vi "Ref_Num_Chart_Generation.vi"(0 "error in (no error)":errorcluster, 1 "Type of Chart":u16(ring) items=[" Crude Semi-Log (Short)", "Crude Semi-Log (Long)", "Bi-directional Crude Semi-Log (Short)", "Bi-directional Crude Semi-Log (Long)"], 2 "Polarity for Max Voltage":u16(ring) items=["Positive", "Negative"], 5 "Start":bool, 6 "Max Voltage":dbl, 10 "CGF_Result T.V.":refnum<vi>, 11 "CGF_START":refnum<vi>, 12 "CGF_error in":refnum<vi>, 14 "CGF_error out":refnum<vi>, 15 "CGF_FINISH":refnum<vi>) -> (4 "error out":errorcluster, 7 "~~ FINISH ~~":bool, 9 "Result - Test Voltages Array":dbl[](array[numeric]))   [LabVIEW 2020]
uses:
  Global 1.vi
panel:
  in  "VRmax":dbl
  in  "x":i32
  out "PositiveVoltages[256]":dbl[](array[numeric])
  out "Checking Value of X":i32
  out "UniD : Test Voltages <OUTPUT>":dbl[](array[numeric])
  in  "SUB SCLC":bool
  out "DONE SUB SCLC":bool
  out "UNIDIRECTIONAL - FINISH Formulating Test Voltages":bool
  in  "SUB LCLC":bool
  out "DONE SUB LCLC":bool
  in  "NumberOfVoltages":i32
  out "NegativeVoltages[256]":dbl[](array[numeric])
  out "Negative value":dbl
  out "Crude Semi-Log (Short)":bool
  out "Crude Semi-Log (Long)":bool
  out "Bi-directional Crude Semi-Log (Short)":bool
  out "Bi-directional Crude Semi-Log (Long)":bool
  out "BIDIRECTIONAL = FINISH Formulating Test Voltages":bool
  in  "SUB Bi-SCLC":bool
  in  "SUB Bi-LCLC":bool
  out "DONE SUB Bi-SCLC":bool
  out "DONE SUB Bi-LCLC":bool
  out "Checking NumberOfVoltages":i32
  out "Flag Formula SCLC":bool
  out "Flag Formula LCLC":bool
  out "first subarray : PosTestV":dbl[](array[numeric])
  out "reversed array : NegTestV":dbl[](array[numeric])
  out "BiD : Test Voltages <OUTPUT>":dbl[](array[numeric])
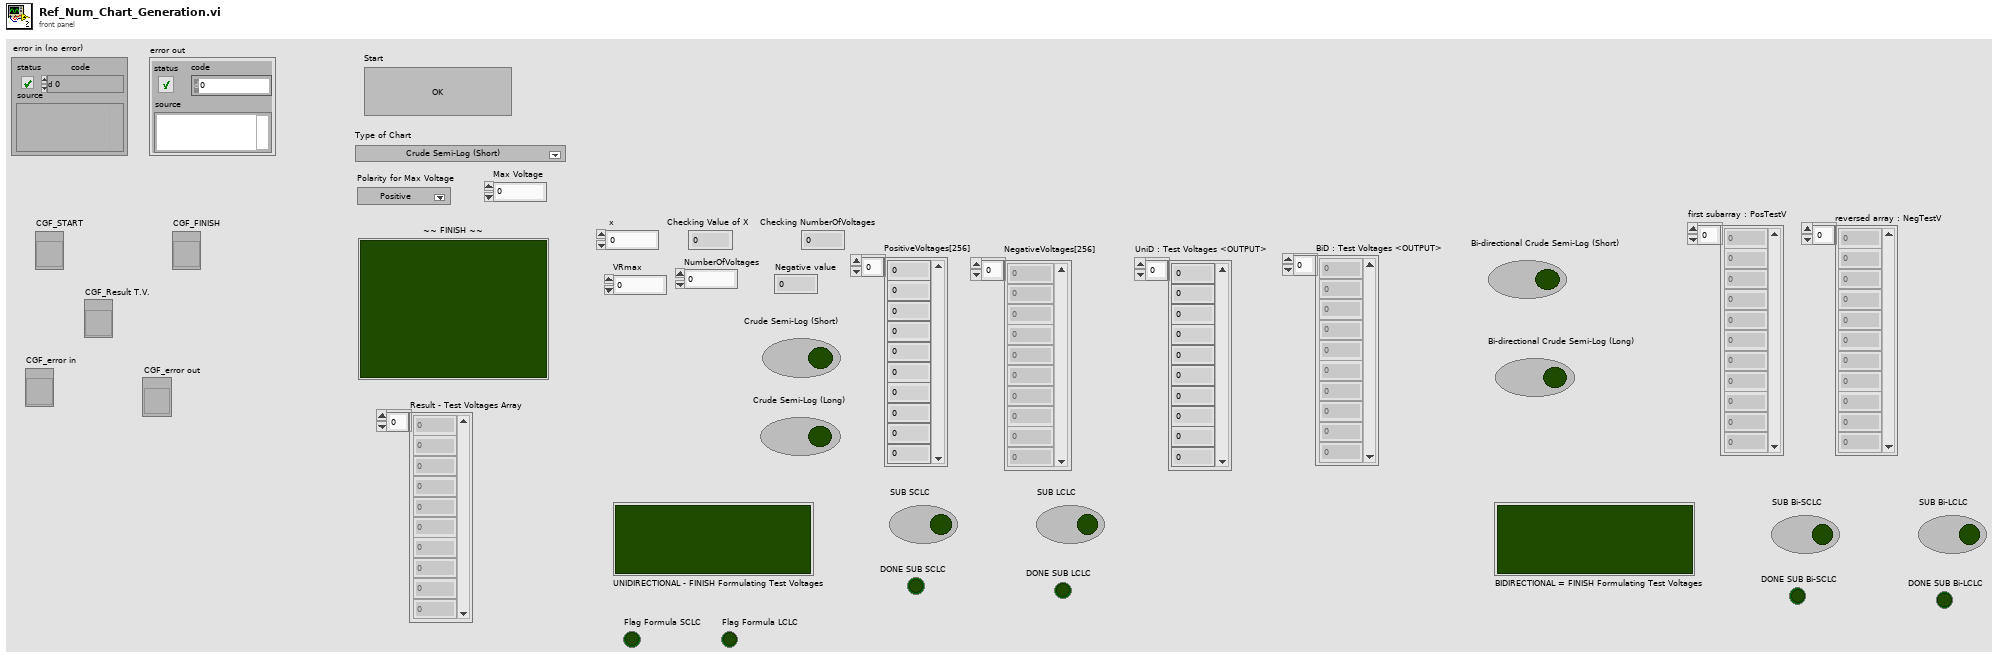
[diagram p1: front panel]
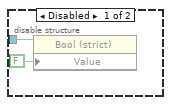
[diagram p2: hidden frame]
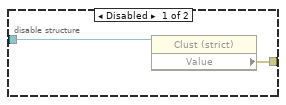
[diagram p3: hidden frame]
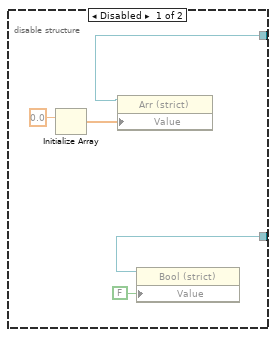
[diagram p4: hidden frame]
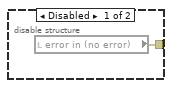
[diagram p5: hidden frame]
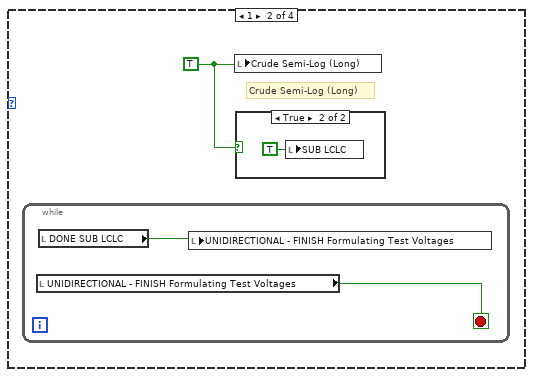
[diagram p7: hidden frame]
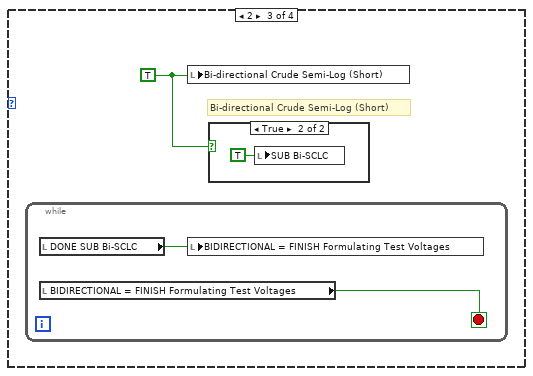
[diagram p9: hidden frame]
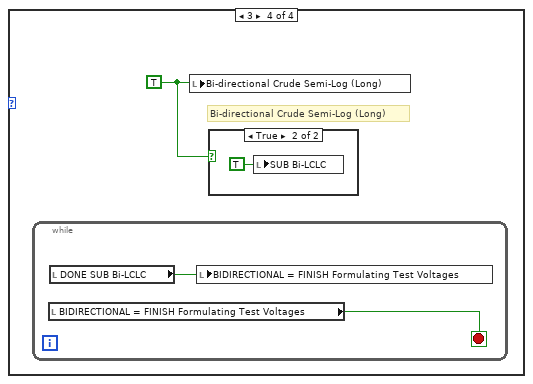
[diagram p11: hidden frame]
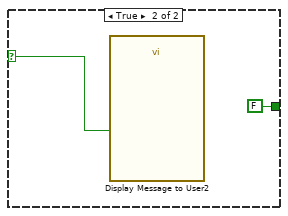
[diagram p16: hidden frame]
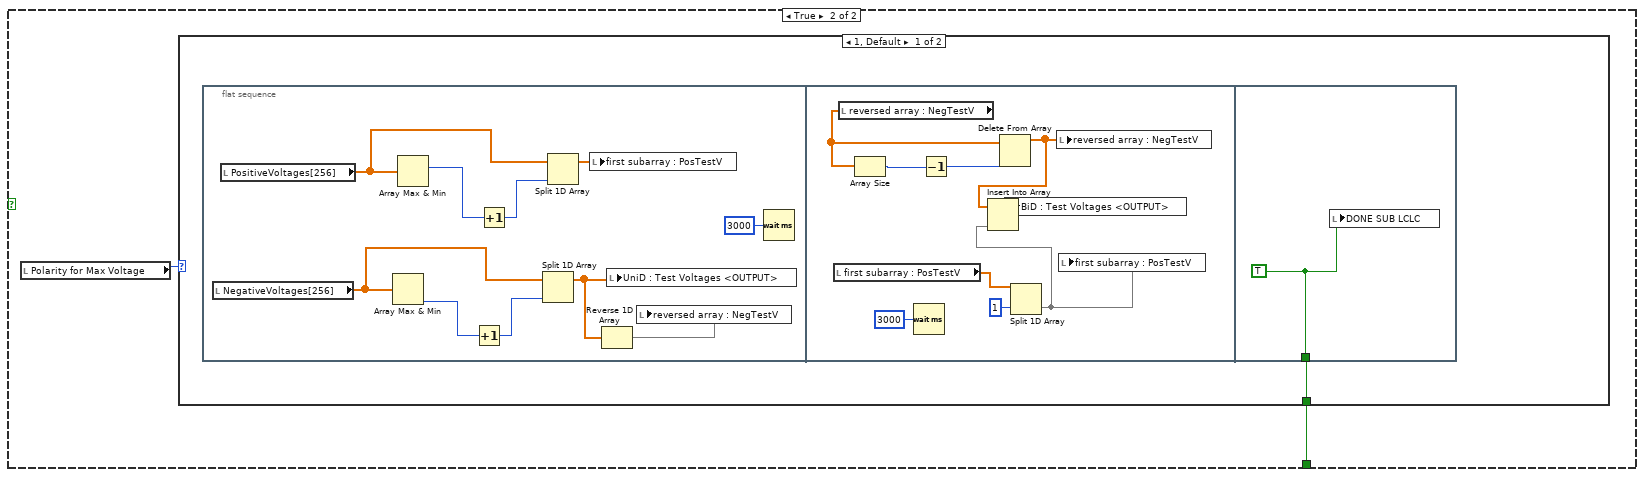
[diagram p17: hidden frame]
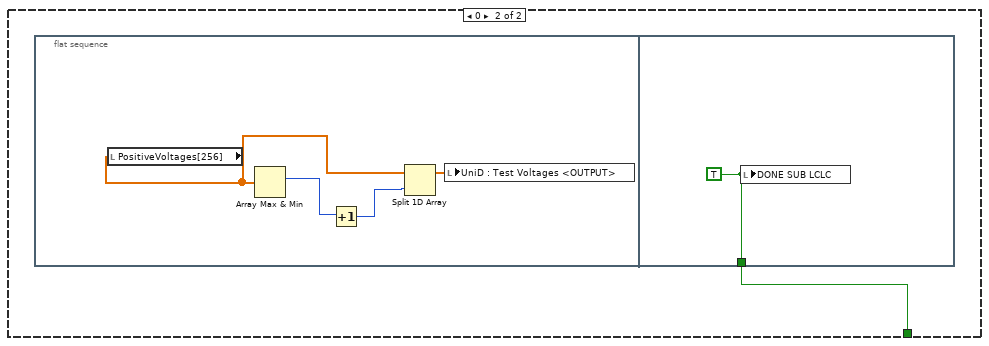
[diagram p18: hidden frame]
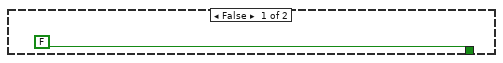
[diagram p19: hidden frame]
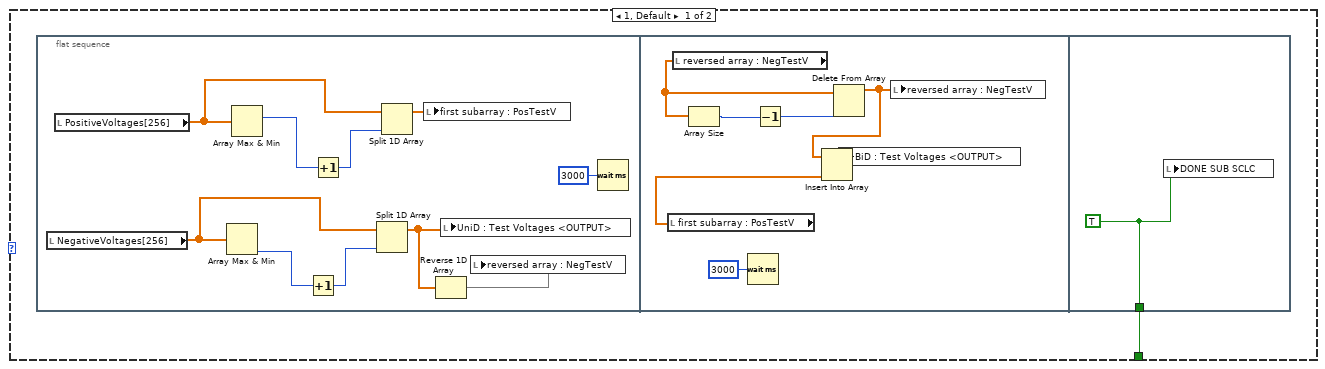
[diagram p20: hidden frame]
diagram:
  n1 = disable-structure shown="Enabled" {
    disable-tunnel: "CGF_error in" -> [w10 _]
    disable-tunnel: "CGF_error out" -> [w9 _]
    disable-tunnel: "CGF_START" -> [w6 _]
    disable-tunnel: "CGF_FINISH" -> [w7 _]
    disable-tunnel: "CGF_Result T.V." -> [w8 _]
    frame Enabled {
      w22 = 0.0
      w11 = FALSE
      # "Bi-directional Crude Semi-Log (Long)"
      # "Bi-directional Crude Semi-Log (Short)"
      # "Initialize"
      # "State Machine of VI"
      # "Error Handler"
      # "Long Sortalog chart bidirectional"
      # "="
      # "Short Sortalog chart bidirectional"
      # "="
      # "="
      # "="
      # "Long Sortalog chart unidirectional"
      # "Short Sortalog chart unidirectional"
      # "Bi-directional Crude Semi-Log (Long)"
      # "Bi-directional Crude Semi-Log (Short)"
      # "Crude Semi-Log (Long)"
      # "Crude Semi-Log (Short)"
      # "DONE :\n\n1) SUB SCLC\n2) SUB SCLC"
      # "ALL VARIABLES"
      # "SUB Function :\nLongCrudeLogChart (VRmax!, Polarity$)"
      # "SUB Function :\n ShortCrudeLogChart (VRmax!, Polarity$)"
      # "Type of Chart :\n\n1) Linear\n2) Crude Semi-Log (Short) \n3) Crude Semi-Log (Long)\n4) Bi-directional Crude Semi-Log (Short)\n5) Bi-directional Crude Semi-Log (Long)"
      # "Linear has been done by Daniel in Generate_Report_NEW\n\nXY Graph : \nArray of X -> Test Voltages\nArray of Y -> Result Arrays"
      n2 = flat-sequence {
        frame #0 {
          n3 = while {
            stop <- w286 stop-if-true
            n4 = local read "SUB SCLC"() -> (w286:bool)
          }
        }
        frame #1 {
          w294 = dbl[] [0.0, 0.1, 0.2, 0.3, 0.4, 0.5, 0.7, 1.0, 2.0, 3.0, 4.0, 5.0, 7.0, 10.0, 20.0, 30.0, 40.0, 50.0, 70.0, 100.0, 200.0]
          # "Bias V"
          n5 = local read "NumberOfVoltages"() -> (w288:i32)
          n6 = Array Max & Min(array=w294) -> (max value=w293:dbl)  [unwired: 3 out]
          n7 = local read "VRmax"() -> (w291:dbl)
          n8 = local read "x"() -> (w292:i32)
          n9 = formula code="// declaration\n\nNumberOfVoltages = 1;\nfloat TestVoltages[256];\n\nx = 1 ;\n//while loop\n\n while   ( VRmax > BiasV[x]  &&  x <= UpBound ) \n {\n\nTestVoltages[x] = BiasV[x];\nx = x + 1;\n}\n//\n\nTestVoltages[x] = VRmax;\nNumberOfVoltages = x;"("x"=w292, "VRmax"=w291, "BiasV"=w294, "NumberOfVoltages"=w288, "UpBound"=w293) -> ("x"=w290:i32, "TestVoltages"=w289:dbl[], "NumberOfVoltages"=w287:i32)
          n10 = local write "PositiveVoltages[256]"(w289) -> ()
          n11 = local write "Checking NumberOfVoltages"(w287) -> ()
          n12 = local write "Checking Value of X"(w290) -> ()
        }
        frame #2 {
          # "If Polarity = 1, then Polarity = Negative"
          # "Create array with negative value for Polarity = Negative"
          n13 = local read "Polarity for Max Voltage"() -> (w295:u16)
          n14 = case shown="0, Default" w295 {
            frame 0, Default {
            }
            frame 1 {
              n15 = local read "PositiveVoltages[256]"() -> (w297:dbl[])
              n16 = Array Size(array=w297) -> (size(s)=w296:i32)
              n17 = for {
                N: w296 -> [_]
                tunnel: w297 -> [w303]
                i -> [w300]
                n18 = Index Array(array=w303, index=w300) -> (element=w304:dbl)
                n19 = Wait (ms)(milliseconds to wait=u32 1000) -> ()  [unwired: 1 out]
                n20 = Negate(x=w304) -> (-x=w301:dbl)
                n21 = local write "Negative value"(w301) -> ()
                n22 = feedback #1() -> (w299:dbl[])  [unwired: 1 in]
                n23 = local write "NegativeVoltages[256]"(w299) -> ()
                n24 = Insert Into Array(array=w299, index=w300, new element=w301) -> (w298:dbl[])
                n25 = feedback-in #1(w298) -> ()
              }
            }
          }
        }
        frame #3 {
          # "Add last element into Negative Array"
          # "If Polarity = 1, then Polarity = Negative"
          n26 = local read "Polarity for Max Voltage"() -> (w305:u16)
          n27 = case shown="0, Default" w305 {
            frame 0, Default {
            }
            frame 1 {
              n28 = local read "NegativeVoltages[256]"() -> (w306:dbl[])
              n29 = Wait (ms)(milliseconds to wait=u32 500) -> ()  [unwired: 1 out]
              n30 = local read "PositiveVoltages[256]"() -> (w309:dbl[])
              n31 = Array Max & Min(array=w309) -> (max index (indices)=w308:i32)  [unwired: 3 out]
              n32 = Index Array(array=w309, index=w308) -> (element=w312:dbl)
              n33 = Negate(x=w312) -> (-x=w310:dbl)
              n34 = local write "Negative value"(w310) -> ()
              n35 = Insert Into Array(array=w306, index=w308, new element=w310) -> (w307:dbl[])
              n36 = local write "NegativeVoltages[256]"(w307) -> ()
            }
          }
        }
        frame #4 {
          # "Replace -0 to 0 in 1st index of array"
          # "If Polarity = 1, then Polarity = Negative"
          n37 = local read "Polarity for Max Voltage"() -> (w313:u16)
          n38 = case shown="0, Default" w313 {
            frame 0, Default {
            }
            frame 1 {
              n39 = local read "NegativeVoltages[256]"() -> (w317:dbl[])
              n40 = Wait (ms)(milliseconds to wait=u32 500) -> ()  [unwired: 1 out]
              n41 = Replace Array Subset(array=w317, new element=0.0 ("new element/subarray"), index=0) -> (w316:dbl[])
              n42 = local write "NegativeVoltages[256]"(w316) -> ()
            }
          }
        }
        frame #5 {
          n43 = local write "Flag Formula SCLC"(TRUE) -> ()
        }
      }
      n44 = while {
        stop <- w162 stop-if-true
        n45 = local read "Flag Formula SCLC"() -> (w163:bool)
        n46 = Wait (ms)(milliseconds to wait=u32 800) -> ()  [unwired: 1 out]
        n47 = case shown="True" w163 {
          tunnel: [FALSE ("FINISH CHART") w166] -> w162
          frame False {
          }
          frame True {
            n48 = local read "Polarity for Max Voltage"() -> (w165:u16)
            n49 = case shown="0" w165 {
              tunnel: [w167 w186] -> w166
              frame 1, Default {
                n50 = flat-sequence {
                  tunnel: [w185] -> w167
                  frame #0 {
                    n51 = local read "NegativeVoltages[256]"() -> (w177:dbl[])
                    n52 = local read "PositiveVoltages[256]"() -> (w171:dbl[])
                    n53 = Array Max & Min(array=w177) -> (min index (indices)=w176:i32)  [unwired: 3 out]
                    n54 = Array Max & Min(array=w171) -> (max index (indices)=w170:i32)  [unwired: 3 out]
                    n55 = Increment(x=w176) -> (x+1=w173:i32)
                    n56 = Increment(x=w170) -> (x+1=w172:i32)
                    n57 = Split 1D Array(array=w177, index=w173) -> (first subarray=w174:dbl[])  [unwired: 1 out]
                    n58 = Split 1D Array(array=w171, index=w172) -> (first subarray=w169:dbl[])  [unwired: 1 out]
                    n59 = local write "first subarray : PosTestV"(w169) -> ()
                    n60 = Reverse 1D Array(array=w174) -> (reversed array=w168:dbl[])
                    n61 = local write "UniD : Test Voltages <OUTPUT>"(w174) -> ()
                    n62 = local write "reversed array : NegTestV"(w168) -> ()
                    n63 = Wait (ms)(milliseconds to wait=u32 3000) -> ()  [unwired: 1 out]
                  }
                  frame #1 {
                    n64 = local read "first subarray : PosTestV"() -> (w184:dbl[])
                    n65 = local read "reversed array : NegTestV"() -> (w182:dbl[])
                    n66 = Array Size(array=w182) -> (size(s)=w181:i32)
                    n67 = Wait (ms)(milliseconds to wait=u32 3000) -> ()  [unwired: 1 out]
                    n68 = Decrement(x=w181) -> (x-1=w180:i32)
                    n69 = Delete From Array(array=w182, index=w180) -> (array with subset deleted=w178:dbl[])  [unwired: 1 in, 1 out]
                    n70 = Insert Into Array(array=w178, new element=w184) -> (w179:dbl[])  [unwired: 1 in]
                    n71 = local write "BiD : Test Voltages <OUTPUT>"(w179) -> ()
                    n72 = local write "reversed array : NegTestV"(w178) -> ()
                  }
                  frame #2 {
                    w185 = TRUE ("FINISH CHART")
                    n73 = local write "DONE SUB SCLC"(w185) -> ()
                  }
                }
              }
              frame 0 {
                n74 = flat-sequence {
                  tunnel: [w191] -> w186
                  frame #0 {
                    n75 = local read "PositiveVoltages[256]"() -> (w188:dbl[])
                    n76 = Array Max & Min(array=w188) -> (max index (indices)=w190:i32)  [unwired: 3 out]
                    n77 = Increment(x=w190) -> (x+1=w189:i32)
                    n78 = Split 1D Array(array=w188, index=w189) -> (first subarray=w187:dbl[])  [unwired: 1 out]
                    n79 = local write "UniD : Test Voltages <OUTPUT>"(w187) -> ()
                  }
                  frame #1 {
                    w191 = TRUE ("FINISH CHART")
                    n80 = local write "DONE SUB SCLC"(w191) -> ()
                  }
                }
              }
            }
          }
        }
      }
      n81 = flat-sequence {
        frame #0 {
          n82 = while {
            stop <- w51 stop-if-true
            n83 = local read "SUB Bi-SCLC"() -> (w51:bool)
          }
        }
        frame #1 {
          w53 = u16 1 items=["Positive", "Negative"] ("Polarity for Max Voltage")
          n84 = local write "Polarity for Max Voltage"(w53) -> ()
          n85 = Wait (ms)(milliseconds to wait=u32 500) -> ()  [unwired: 1 out]
        }
        frame #2 {
          n86 = while {
            stop <- w56 stop-if-true
            n87 = local read "DONE SUB SCLC"() -> (w56:bool)
          }
          n88 = local write "SUB SCLC"(TRUE ("SUB SCLC")) -> ()
          n89 = Wait (ms)(milliseconds to wait=u32 1000) -> ()  [unwired: 1 out]
        }
        frame #3 {
          n90 = local write "DONE SUB Bi-SCLC"(TRUE ("DONE SUB Bi-SCLC")) -> ()
        }
      }
      n91 = while {
        stop <- w118 stop-if-true
        n92 = local read "Max Voltage"() -> (w120:dbl)
        n93 = Equal?(x=w120, y=999.0) -> (x = y?=w123:bool)
        n94 = Equal?(x=w120, y=-999.0) -> (x = y?=w122:bool)
        n95 = Or(x=w123, y=w122) -> (x .or. y?=w119:bool)
        n96 = case shown="False" w119 {
          selector: w119 -> [_ w127]
          tunnel: [TRUE FALSE] -> w118
          frame False {
          }
          frame True {
            n97 = call "Display Message to User2"("Enable"=w127) -> ()  [unwired: 9 in, 2 out]
          }
        }
      }
      n98 = disable-structure shown="Enabled" {
        disable-tunnel: [w43 _] -> _
        frame Disabled {
          n99 = local read "error in (no error)"() -> (w43:errorcluster)
        }
        frame Enabled {
        }
      }
      n100 = disable-structure shown="Enabled" {
        disable-tunnel: w10 -> [w37 _]
        disable-tunnel: [w36 _] -> _
        frame Disabled {
          n101 = property class="Clust (strict)"(reference=w37) -> ("Value"=w36:errorcluster)  [unwired: 1 in, 2 out]
        }
        frame Enabled {
        }
      }
      n102 = flat-sequence {
        tunnel: [w59] -> w33
        tunnel: w6 -> [w58]
        tunnel: [w66] -> w32
        tunnel: w33 -> [w66]
        tunnel: w32 -> [w86]
        tunnel: w9 -> [w91]
        tunnel: w7 -> [w90]
        tunnel: w8 -> [w89]
        frame #0 {
          n103 = while {
            tunnel: [w62] -> w59
            tunnel: w58 -> [w61]
            stop <- w64 stop-if-true
            n104 = local read "error in (no error)"() -> (w60:errorcluster)
            n105 = property class="Bool (strict)"(reference=w61, error in=w60) -> (error out=w62:errorcluster, "Value"=w63:bool)  [unwired: 1 out]
            n106 = local read "Start"() -> (w65:bool)
            n107 = Or(x=w65, y=w63) -> (x .or. y?=w64:bool)
          }
        }
        frame #1 {
          n108 = local read "Type of Chart"() -> (w69:u16)
          n109 = case shown="0, Default" w69 {
            frame 0, Default {
              w70 = TRUE ("Crude Semi-Log (Short)")
              # "Crude Semi-Log (Short)"
              n110 = while {
                stop <- w71 stop-if-true
                n111 = local read "DONE SUB SCLC"() -> (w72:bool)
                n112 = local read "UNIDIRECTIONAL - FINISH Formulating Test Voltages"() -> (w71:bool)
                n113 = local write "UNIDIRECTIONAL - FINISH Formulating Test Voltages"(w72) -> ()
              }
              n114 = local write "Crude Semi-Log (Short)"(w70) -> ()
              n115 = case shown="True" w70 {
                frame False {
                }
                frame True {
                  n116 = local write "SUB SCLC"(TRUE ("SUB SCLC")) -> ()
                }
              }
            }
            frame 1 {
              w74 = TRUE ("Crude Semi-Log (Long)")
              # "Crude Semi-Log (Long)"
              n117 = while {
                stop <- w75 stop-if-true
                n118 = local read "UNIDIRECTIONAL - FINISH Formulating Test Voltages"() -> (w75:bool)
                n119 = local read "DONE SUB LCLC"() -> (w76:bool)
                n120 = local write "UNIDIRECTIONAL - FINISH Formulating Test Voltages"(w76) -> ()
              }
              n121 = local write "Crude Semi-Log (Long)"(w74) -> ()
              n122 = case shown="True" w74 {
                frame False {
                }
                frame True {
                  n123 = local write "SUB LCLC"(TRUE ("SUB SCLC")) -> ()
                }
              }
            }
            frame 2 {
              w78 = TRUE ("Bi-directional Crude Semi-Log (Short)")
              # "Bi-directional Crude Semi-Log (Short)"
              n124 = while {
                stop <- w79 stop-if-true
                n125 = local read "DONE SUB Bi-SCLC"() -> (w80:bool)
                n126 = local read "BIDIRECTIONAL = FINISH Formulating Test Voltages"() -> (w79:bool)
                n127 = local write "BIDIRECTIONAL = FINISH Formulating Test Voltages"(w80) -> ()
              }
              n128 = local write "Bi-directional Crude Semi-Log (Short)"(w78) -> ()
              n129 = case shown="True" w78 {
                frame False {
                }
                frame True {
                  n130 = local write "SUB Bi-SCLC"(TRUE ("SUB Bi-SCLC")) -> ()
                }
              }
            }
            frame 3 {
              w82 = TRUE ("Bi-directional Crude Semi-Log (Long)")
              # "Bi-directional Crude Semi-Log (Long)"
              n131 = while {
                stop <- w83 stop-if-true
                n132 = local read "BIDIRECTIONAL = FINISH Formulating Test Voltages"() -> (w83:bool)
                n133 = local read "DONE SUB Bi-LCLC"() -> (w84:bool)
                n134 = local write "BIDIRECTIONAL = FINISH Formulating Test Voltages"(w84) -> ()
              }
              n135 = local write "Bi-directional Crude Semi-Log (Long)"(w82) -> ()
              n136 = case shown="True" w82 {
                frame False {
                }
                frame True {
                  n137 = local write "SUB Bi-LCLC"(TRUE ("SUB Bi-LCLC")) -> ()
                }
              }
            }
          }
          n138 = call "Display Message to User3"("Message"="<<  START   >>\nInserting Test Voltages") -> ()  [unwired: 9 in, 2 out]
          n139 = Wait (ms)(milliseconds to wait=u32 1000) -> ()  [unwired: 1 out]
        }
        frame #2 {
          n140 = Wait (ms)(milliseconds to wait=u32 800) -> ()  [unwired: 1 out]
          n141 = while {
            tunnel: [w109] -> w93
            tunnel: w89 -> [w106]
            tunnel: [w103] -> w88
            tunnel: w86 -> [w102]
            tunnel: w86 -> [w101]
            stop <- w109 stop-if-true
            n142 = local read "BIDIRECTIONAL = FINISH Formulating Test Voltages"() -> (w107:bool)
            n143 = local read "UNIDIRECTIONAL - FINISH Formulating Test Voltages"() -> (w108:bool)
            n144 = case shown="True" w108 {
              tunnel: w106 -> [_ w117]
              tunnel: [_ w116] -> w105
              tunnel: w102 -> [_ w115]
              frame False {
              }
              frame True {
                n145 = local read "UniD : Test Voltages <OUTPUT>"() -> (w114:dbl[])
                n146 = global write "Global 1.vi" "Result - Test Voltages Array"(w114) -> ()
                n147 = local write "Result - Test Voltages Array"(w114) -> ()
                n148 = property class="Arr (strict)"(reference=w117, error in=w115, "Value"=w114) -> (error out=w116:errorcluster)  [unwired: 1 out]
              }
            }
            n149 = case shown="True" w107 {
              tunnel: w106 -> [_ w113]
              tunnel: [_ w112] -> w104
              tunnel: w101 -> [_ w111]
              frame False {
              }
              frame True {
                n150 = local read "BiD : Test Voltages <OUTPUT>"() -> (w110:dbl[])
                n151 = local write "Result - Test Voltages Array"(w110) -> ()
                n152 = global write "Global 1.vi" "Result - Test Voltages Array"(w110) -> ()
                n153 = property class="Arr (strict)"(reference=w113, error in=w111, "Value"=w110) -> (error out=w112:errorcluster)  [unwired: 1 out]
              }
            }
            n154 = Or(x=w108, y=w107) -> (x .or. y?=w109:bool)
            n155 = Merge Errors(w105, w104) -> (w103:errorcluster)
          }
          n156 = Merge Errors(w88, w86) -> (w87:errorcluster)
          n157 = case shown="True" w93 {
            selector: w93 -> [_ w98]
            tunnel: w87 -> [_ w97]
            tunnel: w91 -> [_ w99]
            tunnel: w90 -> [_ w96]
            frame False {
            }
            frame True {
              n158 = property class="Bool (strict)"(reference=w96, error in=w97, "Value"=w98) -> (error out=w95:errorcluster)  [unwired: 1 out]
              n159 = property class="Clust (strict)"(reference=w99, error in=w95, "Value"=w95) -> (error out=w94:errorcluster)  [unwired: 1 out]
              n160 = local write "~~ FINISH ~~"(w98) -> ()
              n161 = local write "error out"(w94) -> ()
              n162 = call "Display Message to User4"("Enable"=w98, "Message"="<<  DONE  >> \nInserting Test Voltages") -> ()  [unwired: 8 in, 2 out]
            }
          }
        }
      }
      n163 = disable-structure shown="Enabled" {
        disable-tunnel: w6 -> [w35 _]
        frame Disabled {
          n164 = property class="Bool (strict)"(reference=w35, "Value"=FALSE) -> ()  [unwired: 1 in, 2 out]
        }
        frame Enabled {
        }
      }
      n165 = flat-sequence {
        frame #0 {
          n166 = while {
            stop <- w192 stop-if-true
            n167 = local read "SUB LCLC"() -> (w192:bool)
          }
        }
        frame #1 {
          n168 = local read "VRmax"() -> (w194:dbl)
          n169 = Less Or Equal?(x=w194, y=200.0) -> (x <= y?=w195:bool)
          n170 = case shown="True" w195 {
            frame False {
              n171 = Initialize Array(0.0 ("element")) -> (w197:dbl[])  [unwired: 1 in]
              n172 = local write "PositiveVoltages[256]"(w197) -> ()
              n173 = local write "NumberOfVoltages"(1 ("NumberOfVoltages")) -> ()
            }
            frame True {
              n174 = local read "NumberOfVoltages"() -> (w201:i32)
              n175 = local read "VRmax"() -> (w204:dbl)
              n176 = local read "x"() -> (w202:i32)
              n177 = Multiply(x=w204, y=10.0) -> (x*y=w206:dbl)
              n178 = case shown="0..31" w206 {
                tunnel: w204 -> [w213 w217 w225 w232 w239 w246 w253 _]
                tunnel: [w212 w219 w224 w231 w238 w245 w252 _] -> w203
                tunnel: w202 -> [w211 w218 w226 w233 w240 w247 w254 _]
                tunnel: w201 -> [w210 w220 w227 w234 w241 w248 w255 _]
                tunnel: [w208 w215 w222 w229 w236 w243 w250 _] -> w200
                tunnel: [w207 w214 w221 w228 w235 w242 w249 _] -> w199
                frame 0..31 {
                  n179 = formula code="// declaration\n//' Set bias 0 to VRmax! at 0.1V increments (32 voltages)\nNumberOfVoltages = 1;\nfloat TestVoltages[256];\n\nfor (    (x = 0); (x <= VRmax*10); x++   ){\nTestVoltages[x+1] = x / 10;\nNumberOfVoltages = x + 1;\n}"("VRmax"=w213, "x"=w211, "NumberOfVoltages"=w210) -> ("TestVoltages"=w212:dbl[], "x"=w208:i32, "NumberOfVoltages"=w207:i32)
                  n180 = Wait (ms)(milliseconds to wait=u32 500) -> ()  [unwired: 1 out]
                }
                frame 32..100 {
                  n181 = formula code="// declaration\n//'  Set bias 0,.1,.2,.3,.4,.5,.6,.7,.8,.9,1,1.1,1.2,1.5,2,2.5,...s)\nNumberOfVoltages = 1;\nfloat TestVoltages[256];\n//---------------------------------------------\n//---------------------------------------------\nfor (    (x = 0); (x <=11); x++   ){\nTestVoltages[x+1] = x / 10;\n}\n//---------------------------------------------\nTestVoltages[13] = 1.3;\nTestVoltages[14] = 1.5;\n//---------------------------------------------\nfor (    (x = 4); (x <= VRmax*2); x++   ){\nTestVoltages[11+x] = x / 2;\nNumberOfVoltages =11+x;\n}\n//---------------------------------------------\nTestVoltages[NumberOfVoltages] = abs(VRmax);"("VRmax"=w217, "x"=w218, "NumberOfVoltages"=w220) -> ("TestVoltages"=w219:dbl[], "x"=w215:i32, "NumberOfVoltages"=w214:i32)
                  n182 = Wait (ms)(milliseconds to wait=u32 500) -> ()  [unwired: 1 out]
                }
                frame 101..199 {
                  n183 = formula code="// declaration\n//'  Set bias 0,.1,.2,.3,.4,.5,.6,.7,.8,.9,1,1.1,1.3,1.5,2,3,...\nNumberOfVoltages = 1;\nfloat TestVoltages[256];\n//---------------------------------------------\n//---------------------------------------------\nfor (    (x = 0); (x <=11); x++   ){\nTestVoltages[x+1] = x / 10;\n}\n//---------------------------------------------\nTestVoltages[13] = 1.3;\nTestVoltages[14] = 1.5;\n//---------------------------------------------\nfor (    (x = 2); (x <= int(VRmax)); x++   ){\nTestVoltages[13+x] = x;\nNumberOfVoltages =13+x;\n}\n//---------------------------------------------\nTestVoltages[NumberOfVoltages] = abs(VRmax);"("VRmax"=w225, "x"=w226, "NumberOfVoltages"=w227) -> ("TestVoltages"=w224:dbl[], "x"=w222:i32, "NumberOfVoltages"=w221:i32)
                  n184 = Wait (ms)(milliseconds to wait=u32 500) -> ()  [unwired: 1 out]
                }
                frame 200..300 {
                  n185 = formula code="// declaration\n//'  Set bias 0,.1,.2,.3,.4,.5,.6,.7,.8,.9,1,1.1,1.3,1.5,2,3,...\nNumberOfVoltages = 1;\nfloat TestVoltages[256];\n//---------------------------------------------\n//---------------------------------------------\nfor (    (x = 0); (x<=11); x++   ){\nTestVoltages[x+1] = x / 10;\n}\n//---------------------------------------------\nTestVoltages[13] = 1.3;\nTestVoltages[14] = 1.5;\n//---------------------------------------------\nfor (    (x = 2); (x <= int(VRmax)); x=x+2   ){\nTestVoltages[14+ x/2] = x;\nNumberOfVoltages =14+ x/2;\n}\n//---------------------------------------------\nTestVoltages[NumberOfVoltages] = abs(VRmax);"("VRmax"=w232, "x"=w233, "NumberOfVoltages"=w234) -> ("TestVoltages"=w231:dbl[], "x"=w229:i32, "NumberOfVoltages"=w228:i32)
                  n186 = Wait (ms)(milliseconds to wait=u32 500) -> ()  [unwired: 1 out]
                }
                frame 301..350 {
                  n187 = formula code="// declaration\n//'  Set bias 0,.1,.2,.3,.4,.5,.6,.7,.8,.9,1,1.1,1.3,1.5,2,5,10,...\nNumberOfVoltages = 1;\nfloat TestVoltages[256];\n//---------------------------------------------\n//---------------------------------------------\nfor (    (x = 0); (x <=11); x++   ){\nTestVoltages[x+1] = x / 10;\n}\n//---------------------------------------------\nTestVoltages[13] = 1.3;\nTestVoltages[14] = 1.5;\nTestVoltages[15] = 2;\n//---------------------------------------------\nfor (    (x =5); (x <= int(VRmax)); x=x+5   ){\nTestVoltages[15+ x/5] = x;\nNumberOfVoltages =15+ x/5;\n}\n//---------------------------------------------\nTestVoltages[NumberOfVoltages] = abs(VRmax);"("VRmax"=w239, "x"=w240, "NumberOfVoltages"=w241) -> ("TestVoltages"=w238:dbl[], "x"=w236:i32, "NumberOfVoltages"=w235:i32)
                  n188 = Wait (ms)(milliseconds to wait=u32 500) -> ()  [unwired: 1 out]
                }
                frame 351..1000 {
                  n189 = Wait (ms)(milliseconds to wait=u32 500) -> ()  [unwired: 1 out]
                  n190 = formula code="// declaration\n//'  Set bias 0,.1,.2,.3,.4,.5,.6,.7,.8,.9,1,1.1,1.3,1.5,2,5,10,...\nNumberOfVoltages = 1;\nfloat TestVoltages[256];\n//---------------------------------------------\n//---------------------------------------------\nfor (    (x = 0); (x <=11); x++   ){\nTestVoltages[x+1] = x / 10;\n}\n//---------------------------------------------\nTestVoltages[13] = 1.3;\nTestVoltages[14] = 1.5;\nTestVoltages[15] = 2;\nTestVoltages[16] = 5;\nTestVoltages[17] = 10;\n//---------------------------------------------\nfor (    (x =20); (x <= int(VRmax)); x=x+10  ){\nTestVoltages[16+ x/10] = x;\nNumberOfVoltages =16+ x/10;\n}\n//---------------------------------------------\nTestVoltages[NumberOfVoltages] = abs(VRmax);"("VRmax"=w246, "x"=w247, "NumberOfVoltages"=w248) -> ("TestVoltages"=w245:dbl[], "x"=w243:i32, "NumberOfVoltages"=w242:i32)
                }
                frame 1001..2000 {
                  n191 = Wait (ms)(milliseconds to wait=u32 500) -> ()  [unwired: 1 out]
                  n192 = formula code="// declaration\n//'  Set bias 0,.1,.2,.3,.4,.5,.6,.7,.8,.9,1,1.1,1.3,1.5,2,5,10,...\nNumberOfVoltages = 1;\nfloat TestVoltages[256];\n//---------------------------------------------\n//---------------------------------------------\nfor (    (x = 0); (x <=11); x++   ){\nTestVoltages[x+1] = x / 10;\n}\n//---------------------------------------------\nTestVoltages[13] = 1.3;\nTestVoltages[14] = 1.5;\nTestVoltages[15] = 2;\nTestVoltages[16] = 5;\nTestVoltages[17] = 10;\nTestVoltages[18] = 20;\n//---------------------------------------------\nfor (    (x =20); (x <= int(VRmax)); x=x+20  ){\nTestVoltages[17+ x/20] = x;\nNumberOfVoltages =17+ x/20;\n}\n//---------------------------------------------\nTestVoltages[NumberOfVoltages] = abs(VRmax);"("VRmax"=w253, "x"=w254, "NumberOfVoltages"=w255) -> ("TestVoltages"=w252:dbl[], "x"=w250:i32, "NumberOfVoltages"=w249:i32)
                }
                frame 2001.., Default {
                  n193 = call "Display Message to User"() -> ()  [unwired: 10 in, 2 out]
                }
              }
              n194 = local write "PositiveVoltages[256]"(w203) -> ()
              n195 = local write "Checking NumberOfVoltages"(w199) -> ()
              n196 = local write "Checking Value of X"(w200) -> ()
            }
          }
        }
        frame #2 {
          # "If Polarity = 1, then Polarity = Negative"
          # "Create array with negative value for Polarity = Negative"
          n197 = local read "Polarity for Max Voltage"() -> (w256:u16)
          n198 = case shown="1" w256 {
            frame 0, Default {
            }
            frame 1 {
              n199 = local read "PositiveVoltages[256]"() -> (w258:dbl[])
              n200 = Array Size(array=w258) -> (size(s)=w257:i32)
              n201 = for {
                N: w257 -> [_]
                tunnel: w258 -> [w264]
                i -> [w262]
                n202 = Index Array(array=w264, index=w262) -> (element=w265:dbl)
                n203 = Wait (ms)(milliseconds to wait=u32 1000) -> ()  [unwired: 1 out]
                n204 = Negate(x=w265) -> (-x=w259:dbl)
                n205 = local write "Negative value"(w259) -> ()
                n206 = feedback #2() -> (w260:dbl[])  [unwired: 1 in]
                n207 = local write "NegativeVoltages[256]"(w260) -> ()
                n208 = Insert Into Array(array=w260, index=w262, new element=w259) -> (w261:dbl[])
                n209 = feedback-in #2(w261) -> ()
              }
            }
          }
        }
        frame #3 {
          # "Add last element into Negative Array"
          # "If Polarity = 1, then Polarity = Negative"
          n210 = local read "Polarity for Max Voltage"() -> (w266:u16)
          n211 = case shown="1" w266 {
            frame 0, Default {
            }
            frame 1 {
              n212 = local read "NegativeVoltages[256]"() -> (w267:dbl[])
              n213 = Wait (ms)(milliseconds to wait=u32 500) -> ()  [unwired: 1 out]
              n214 = local read "PositiveVoltages[256]"() -> (w270:dbl[])
              n215 = Array Max & Min(array=w270) -> (max index (indices)=w269:i32)  [unwired: 3 out]
              n216 = Index Array(array=w270, index=w269) -> (element=w273:dbl)
              n217 = Negate(x=w273) -> (-x=w271:dbl)
              n218 = local write "Negative value"(w271) -> ()
              n219 = Insert Into Array(array=w267, index=w269, new element=w271) -> (w268:dbl[])
              n220 = local write "NegativeVoltages[256]"(w268) -> ()
            }
          }
        }
        frame #4 {
          # "Delete first Zero in Both of the Array"
          # "If Polarity = 1, then Polarity = Negative"
          n221 = local read "Polarity for Max Voltage"() -> (w274:u16)
          n222 = case shown="1" w274 {
            frame 0, Default {
            }
            frame 1 {
              n223 = local read "NegativeVoltages[256]"() -> (w277:dbl[])
              n224 = Wait (ms)(milliseconds to wait=u32 500) -> ()  [unwired: 1 out]
              n225 = Delete From Array(array=w277, index=0) -> (array with subset deleted=w276:dbl[])  [unwired: 1 in, 1 out]
              n226 = local write "NegativeVoltages[256]"(w276) -> ()
            }
          }
        }
        frame #5 {
          # "Replace -0 to 0 in 1st index of array"
          # "If Polarity = 1, then Polarity = Negative"
          n227 = local read "Polarity for Max Voltage"() -> (w279:u16)
          n228 = case shown="1" w279 {
            frame 0, Default {
            }
            frame 1 {
              n229 = local read "NegativeVoltages[256]"() -> (w283:dbl[])
              n230 = Wait (ms)(milliseconds to wait=u32 500) -> ()  [unwired: 1 out]
              n231 = Replace Array Subset(array=w283, new element=0.0 ("new element/subarray"), index=0) -> (w282:dbl[])
              n232 = local write "NegativeVoltages[256]"(w282) -> ()
            }
          }
        }
        frame #6 {
          n233 = local write "Flag Formula LCLC"(TRUE ("DONE SUB LCLC")) -> ()
        }
      }
      n234 = while {
        stop <- w129 stop-if-true
        n235 = local read "Flag Formula LCLC"() -> (w130:bool)
        n236 = Wait (ms)(milliseconds to wait=u32 800) -> ()  [unwired: 1 out]
        n237 = case shown="False" w130 {
          tunnel: [FALSE ("FINISH CHART") w133] -> w129
          frame False {
          }
          frame True {
            n238 = local read "Polarity for Max Voltage"() -> (w132:u16)
            n239 = case shown="1, Default" w132 {
              tunnel: [w134 w155] -> w133
              frame 1, Default {
                n240 = flat-sequence {
                  tunnel: [w154] -> w134
                  frame #0 {
                    n241 = local read "NegativeVoltages[256]"() -> (w144:dbl[])
                    n242 = local read "PositiveVoltages[256]"() -> (w138:dbl[])
                    n243 = Array Max & Min(array=w144) -> (min index (indices)=w143:i32)  [unwired: 3 out]
                    n244 = Array Max & Min(array=w138) -> (max index (indices)=w137:i32)  [unwired: 3 out]
                    n245 = Increment(x=w143) -> (x+1=w140:i32)
                    n246 = Increment(x=w137) -> (x+1=w139:i32)
                    n247 = Split 1D Array(array=w144, index=w140) -> (first subarray=w141:dbl[])  [unwired: 1 out]
                    n248 = Split 1D Array(array=w138, index=w139) -> (first subarray=w136:dbl[])  [unwired: 1 out]
                    n249 = local write "first subarray : PosTestV"(w136) -> ()
                    n250 = Reverse 1D Array(array=w141) -> (reversed array=w135:dbl[])
                    n251 = local write "UniD : Test Voltages <OUTPUT>"(w141) -> ()
                    n252 = local write "reversed array : NegTestV"(w135) -> ()
                    n253 = Wait (ms)(milliseconds to wait=u32 3000) -> ()  [unwired: 1 out]
                  }
                  frame #1 {
                    n254 = local read "first subarray : PosTestV"() -> (w147:dbl[])
                    n255 = local read "reversed array : NegTestV"() -> (w152:dbl[])
                    n256 = Array Size(array=w152) -> (size(s)=w151:i32)
                    n257 = Wait (ms)(milliseconds to wait=u32 3000) -> ()  [unwired: 1 out]
                    n258 = Decrement(x=w151) -> (x-1=w150:i32)
                    n259 = Delete From Array(array=w152, index=w150) -> (array with subset deleted=w148:dbl[])  [unwired: 1 in, 1 out]
                    n260 = Split 1D Array(array=w147, index=1) -> (second subarray=w145:dbl[])  [unwired: 1 out]
                    n261 = Insert Into Array(array=w148, new element=w145) -> (w149:dbl[])  [unwired: 1 in]
                    n262 = local write "BiD : Test Voltages <OUTPUT>"(w149) -> ()
                    n263 = local write "reversed array : NegTestV"(w148) -> ()
                    n264 = local write "first subarray : PosTestV"(w145) -> ()
                  }
                  frame #2 {
                    w154 = TRUE ("FINISH CHART")
                    n265 = local write "DONE SUB LCLC"(w154) -> ()
                  }
                }
              }
              frame 0 {
                n266 = flat-sequence {
                  tunnel: [w160] -> w155
                  frame #0 {
                    n267 = local read "PositiveVoltages[256]"() -> (w157:dbl[])
                    n268 = Array Max & Min(array=w157) -> (max index (indices)=w159:i32)  [unwired: 3 out]
                    n269 = Increment(x=w159) -> (x+1=w158:i32)
                    n270 = Split 1D Array(array=w157, index=w158) -> (first subarray=w156:dbl[])  [unwired: 1 out]
                    n271 = local write "UniD : Test Voltages <OUTPUT>"(w156) -> ()
                  }
                  frame #1 {
                    w160 = TRUE ("FINISH CHART")
                    n272 = local write "DONE SUB LCLC"(w160) -> ()
                  }
                }
              }
            }
          }
        }
      }
      n273 = local write "error in (no error)"(errorcluster {"status"=FALSE, "code"=0, "source"=""} ("error in (no error)")) -> ()
      n274 = flat-sequence {
        frame #0 {
          n275 = while {
            stop <- w44 stop-if-true
            n276 = local read "SUB Bi-LCLC"() -> (w44:bool)
          }
        }
        frame #1 {
          w46 = u16 1 items=["Positive", "Negative"] ("Polarity for Max Voltage")
          n277 = local write "Polarity for Max Voltage"(w46) -> ()
          n278 = Wait (ms)(milliseconds to wait=u32 500) -> ()  [unwired: 1 out]
        }
        frame #2 {
          n279 = while {
            stop <- w49 stop-if-true
            n280 = local read "DONE SUB LCLC"() -> (w49:bool)
          }
          n281 = local write "SUB LCLC"(TRUE ("SUB SCLC")) -> ()
          n282 = Wait (ms)(milliseconds to wait=u32 1000) -> ()  [unwired: 1 out]
        }
        frame #3 {
          n283 = local write "DONE SUB Bi-LCLC"(TRUE ("DONE SUB Bi-SCLC")) -> ()
        }
      }
      n284 = local write "error out"(errorcluster {"status"=FALSE, "code"=0, "source"=""} ("error out")) -> ()
      n285 = local write "Start"(w11) -> ()
      n286 = local write "Flag Formula LCLC"(w11) -> ()
      n287 = local write "Flag Formula SCLC"(w11) -> ()
      n288 = local write "Bi-directional Crude Semi-Log (Short)"(w11) -> ()
      n289 = local write "Bi-directional Crude Semi-Log (Long)"(w11) -> ()
      n290 = local write "Crude Semi-Log (Short)"(w11) -> ()
      n291 = local write "Crude Semi-Log (Long)"(w11) -> ()
      n292 = local write "SUB SCLC"(w11) -> ()
      n293 = local write "DONE SUB SCLC"(w11) -> ()
      n294 = local write "SUB LCLC"(w11) -> ()
      n295 = local write "DONE SUB LCLC"(w11) -> ()
      n296 = local write "UNIDIRECTIONAL - FINISH Formulating Test Voltages"(w11) -> ()
      n297 = local write "SUB Bi-SCLC"(w11) -> ()
      n298 = local write "DONE SUB Bi-SCLC"(w11) -> ()
      n299 = local write "BIDIRECTIONAL = FINISH Formulating Test Voltages"(w11) -> ()
      n300 = local write "SUB Bi-LCLC"(w11) -> ()
      n301 = local write "DONE SUB Bi-LCLC"(w11) -> ()
      n302 = local write "~~ FINISH ~~"(w11) -> ()
      n303 = Wait (ms)(milliseconds to wait=u32 1000) -> ()  [unwired: 1 out]
      n304 = local read "Max Voltage"() -> (w29:dbl)
      n305 = Initialize Array(0.0 ("element")) -> (w26:dbl[])  [unwired: 1 in]
      n306 = Initialize Array(0.0 ("element")) -> (w27:dbl[])  [unwired: 1 in]
      n307 = Initialize Array(0.0 ("element")) -> (w25:dbl[])  [unwired: 1 in]
      n308 = Initialize Array(0.0 ("element")) -> (w16:dbl[])  [unwired: 1 in]
      n309 = Initialize Array(0.0 ("element")) -> (w17:dbl[])  [unwired: 1 in]
      n310 = local write "PositiveVoltages[256]"(w25) -> ()
      n311 = local write "UniD : Test Voltages <OUTPUT>"(w26) -> ()
      n312 = Initialize Array(0.0 ("element")) -> (w31:dbl[])  [unwired: 1 in]
      n313 = local write "NegativeVoltages[256]"(w27) -> ()
      n314 = Initialize Array(0.0 ("element")) -> (w30:dbl[])  [unwired: 1 in]
      n315 = Absolute Value(x=w29) -> (abs(x)=w28:dbl)
      n316 = local write "BiD : Test Voltages <OUTPUT>"(w17) -> ()
      n317 = local write "Result - Test Voltages Array"(w16) -> ()
      n318 = local write "Checking NumberOfVoltages"(w22) -> ()
      n319 = local write "Negative value"(w22) -> ()
      n320 = local write "first subarray : PosTestV"(w31) -> ()
      n321 = local write "reversed array : NegTestV"(w30) -> ()
      n322 = local write "Checking Value of X"(w22) -> ()
      n323 = local write "VRmax"(w28) -> ()
      n324 = disable-structure shown="Enabled" {
        disable-tunnel: w8 -> [w42 _]
        disable-tunnel: w7 -> [w39 _]
        frame Disabled {
          n325 = Initialize Array(0.0 ("element")) -> (w40:dbl[])  [unwired: 1 in]
          n326 = property class="Arr (strict)"(reference=w42, "Value"=w40) -> ()  [unwired: 1 in, 2 out]
          n327 = property class="Bool (strict)"(reference=w39, "Value"=FALSE) -> ()  [unwired: 1 in, 2 out]
        }
        frame Enabled {
        }
      }
    }
    frame Disabled {
    }
  }
